vi "read_diag.vi"(10 "Address":u16, 11 "VISA resource name":refnum<visa-resource-name>) -> (1 "timeout":bool, 2 "diag":T1, 3 "VISA resource name out":refnum<visa-resource-name>)   [LabVIEW 2014]
uses:
  controls/diag.ctl
panel:
  out "error out 2":errorcluster
  out "error out":errorcluster
  out "unsigned byte array":u8[](array[numeric])
  out "x+y":u32
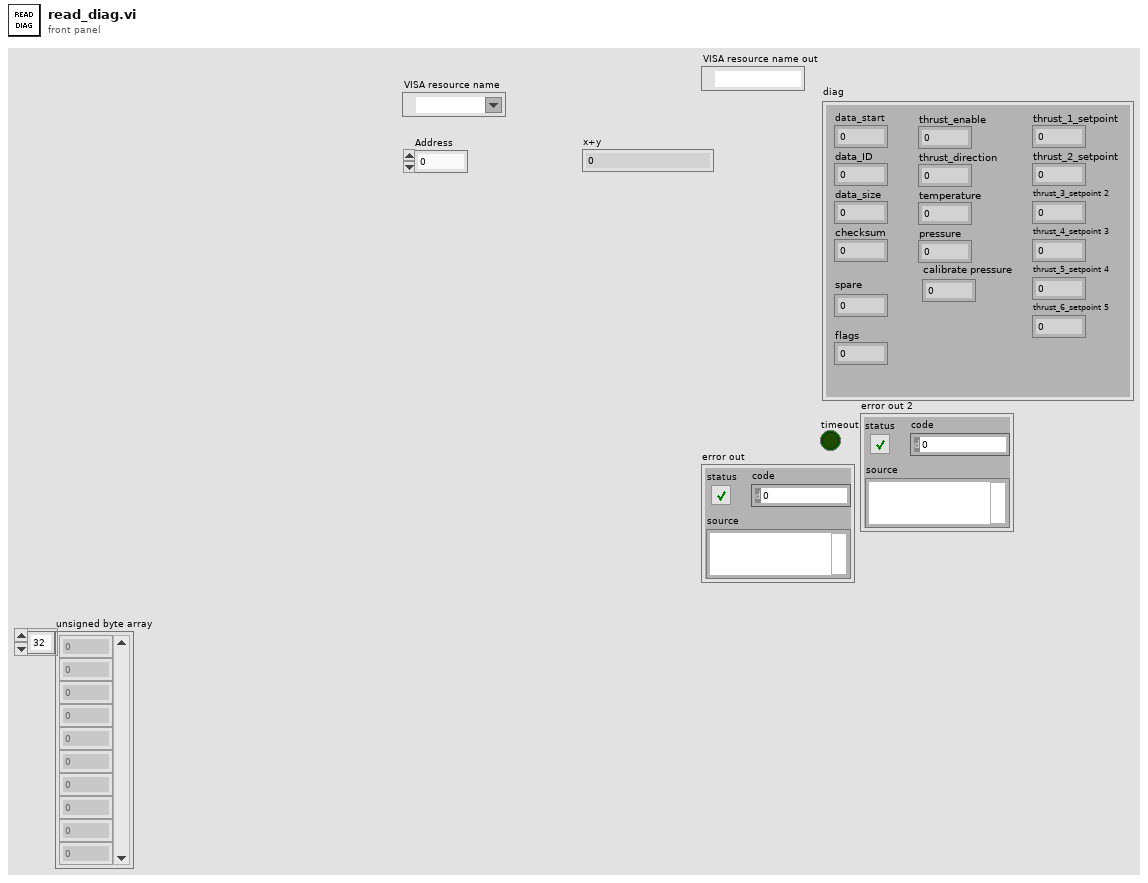
[diagram p1: front panel]
types:
  T1 = typedef "diag.ctl" = cluster{"data_start":u16, "data_ID":u16, "data_size":u16, "thrust_enable":u8, "thrust_direction":u8, "temperature":sgl, "pressure":sgl, "thrust_1_setpoint":u16, "thrust_2_setpoint":u16, "thrust_3_setpoint 2":u16, "thrust_4_setpoint 3":u16, "thrust_5_setpoint 4":u16, "thrust_6_setpoint 5":u16, "spare":u16, "flags":u16, "calibrate pressure":sgl, "checksum":u16}
  T2 = enum16{"big-endian, network order", "native, host order", "little-endian"}
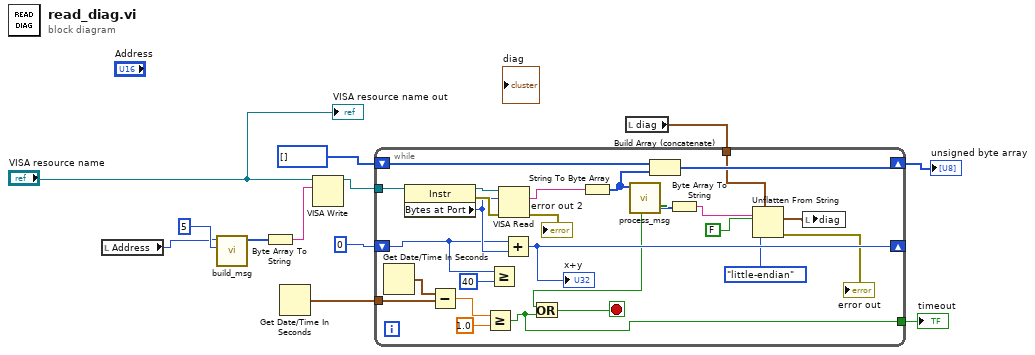
[diagram p0: block diagram]
diagram:
  n1 = local read "Address"() -> (w9:u16)
  n2 = call "build_msg.vi"("ID"=u16 5 ("Address"), "Address"=w9) -> ("msg"=w11:u8[])  [unwired: 9 in]
  n3 = Byte Array To String(unsigned byte array=w11) -> (string=w12:string)
  n4 = Get Date/Time In Seconds() -> (seconds since 1Jan1904=w6:timestamp)
  n5 = VISA Write(VISA resource name="VISA resource name", write buffer=w12) -> (VISA resource name out=w8:refnum<visa-resource-name>)  [unwired: 1 in, 2 out]
  n6 = local read "diag"() -> (w2:T1)
  n7 = while {
    tunnel: w8 -> [w38]
    shift-right: [w37] -> _
    shift-left: u16 0 ("Address") -> [w33]
    tunnel: w6 -> [w30]
    shift-right: [w23] -> w4
    shift-left: u8[] [] ("unsigned byte array") -> [w25]
    tunnel: w2 -> [w19]
    tunnel: [w15] -> w1
    stop <- w27 stop-if-true
    n8 = Get Date/Time In Seconds() -> (seconds since 1Jan1904=w31:timestamp)
    n9 = property class="Instr"(reference=w38) -> (reference out=w35:refnum<visa-resource-name>, error out=w36:errorcluster, "Bytes at Port"=w34:u32)  [unwired: 1 in]
    n10 = Subtract(x=w31, y=w30) -> (x-y=w29:dbl)
    n11 = Greater Or Equal?(x=w29, y=1.0) -> (x >= y?=w15:bool)
    n12 = Greater Or Equal?(x=w33, y=u32 40) -> ()  [unwired: 1 out]
    n13 = VISA Read(VISA resource name=w35, byte count=w34, error in (no error)=w36) -> (read buffer=w26:string, error out=→"error out 2":errorcluster)  [unwired: 2 out]
    n14 = Add(x=w33, y=w34) -> (x+y=w37:u32)
    "x+y" <- w37
    n15 = String To Byte Array(string=w26) -> (unsigned byte array=w24:u8[])
    n16 = call "process_msg.vi"("data"=w24) -> ("valid"=w22:bool, "data_out"=w20:u8[])  [unwired: 6 in, 3 out]
    n17 = Or(x=w22, y=w15) -> (x .or. y?=w27:bool)
    n18 = Build Array (concatenate)(w25, w24) -> (w23:u8[])
    n19 = Byte Array To String(unsigned byte array=w20) -> (string=w21:string)
    n20 = Unflatten From String(type=w19, binary string=w21, data includes array or string size? (T)=FALSE, byte order (0:big-endian, network order)=T2."little-endian") -> (value=w18:T1, error out=→"error out":errorcluster)  [unwired: 1 in, 1 out]
    n21 = local write "diag"(w18) -> ()
  }
  "unsigned byte array" <- w4
  "timeout" <- w1
  "VISA resource name out" <- "VISA resource name"
